vi "Do.vi"(8 "error in (no error)":errorcluster, 10 "Actor in":refnum<class "Actor.lvclass">, 11 "RegisterAppenderMsg":refnum<class "RegisterAppenderMsg.lvclass">) -> (0 "error out":errorcluster, 2 "Actor out":refnum<class "Actor.lvclass">)   [LabVIEW 2026, in "Lumberjack.lvlib" / "RegisterAppenderMsg.lvclass"]
doc: "<p>(<strong>Filename</strong>: <span class=\"dnl\">Actor Framework.lvlib:Message.lvclass:Do.vi</span>)</p>\n<p>Defines what a message does when it is received by an actor. Generally, a message instructs an actor to invoke one of its methods. By default, this method does nothing. A child class must override it to define behavior.</p>"
uses:
  RegisterAppenderMsg.lvclass
  <vilib>/ActorFramework/Actor/Actor.lvclass
  LogManager/LogManager.lvclass/LogManager.lvclass
  C:/Program Files (x86)/National Instruments/LabVIEW 2026/vi.lib/ActorFramework/Actor/Actor.lvclass
  RegisterAppenderMsg.lvclass/RegisterAppenderMsg.ctl
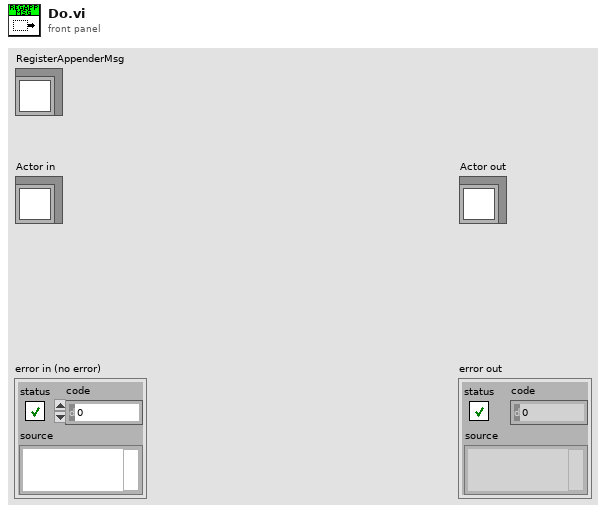
[diagram p1: front panel]
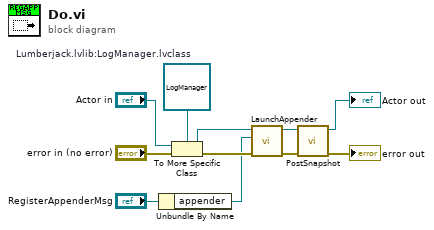
[diagram p0: block diagram]
diagram:
  w10 = refnum<class "LogManager.lvclass"> refnum  # Lumberjack.lvlib:LogManager.lvclass
  n1 = Unbundle By Name("RegisterAppenderMsg") -> ("appender"=w5:refnum<class "Appender.lvclass">)
  n2 = To More Specific Class(target class=w10, reference="Actor in", error in="error in (no error)") -> (specific class reference=w6:refnum<class "LogManager.lvclass">, error out=w7:errorcluster)
  n3 = call "LaunchAppender.vi"("error in (no error)"=w7, "Lumberjack.lvlib:Appender.lvclass"=w5, "LogManager in"=w6) -> ("error out"=w4:errorcluster, "LogManager out"=w3:refnum<class "LogManager.lvclass">)  [unwired: 7 in]
  n4 = call "PostSnapshot.vi"("error in (no error)"=w4, "LogManager in"=w3) -> ("error out"=→"error out":errorcluster, "LogManager out"=→"Actor out":refnum<class "LogManager.lvclass">)  [unwired: 8 in]
